vi "FTW-Actor-LocalMessage-Worker.vi"(0 "FTW-ActorInstance In":refnum<class "FTW-ActorInstance.lvclass">, 5 "Message Header":string, 7 "Message Body":string, 9 "Send Rate":dbl, 11 "error in":errorcluster, 12 "Lossless (F)":bool, 14 "max queue size (1)":i32=1) -> ()   [LabVIEW 2013, in "FTW-ActorInstance.lvclass"]
uses:
  FTW-ActorInstance.lvclass
  FTW-ActorInstance.lvclass/FTW-ActorInstance.ctl
  Message/Base/FTW-Message.lvclass
  Message/Lossy/FTW-Message-Lossy.lvclass
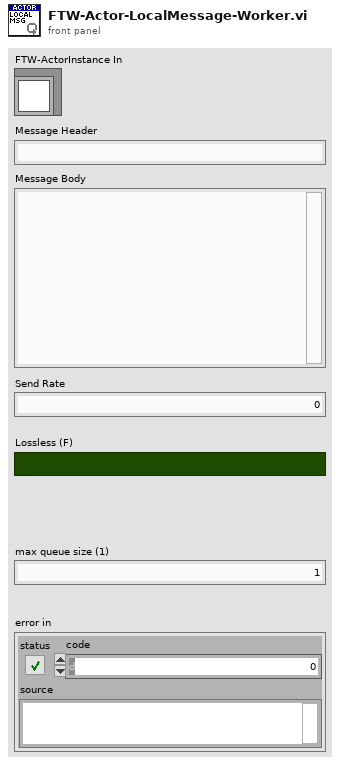
[diagram p1: front panel]
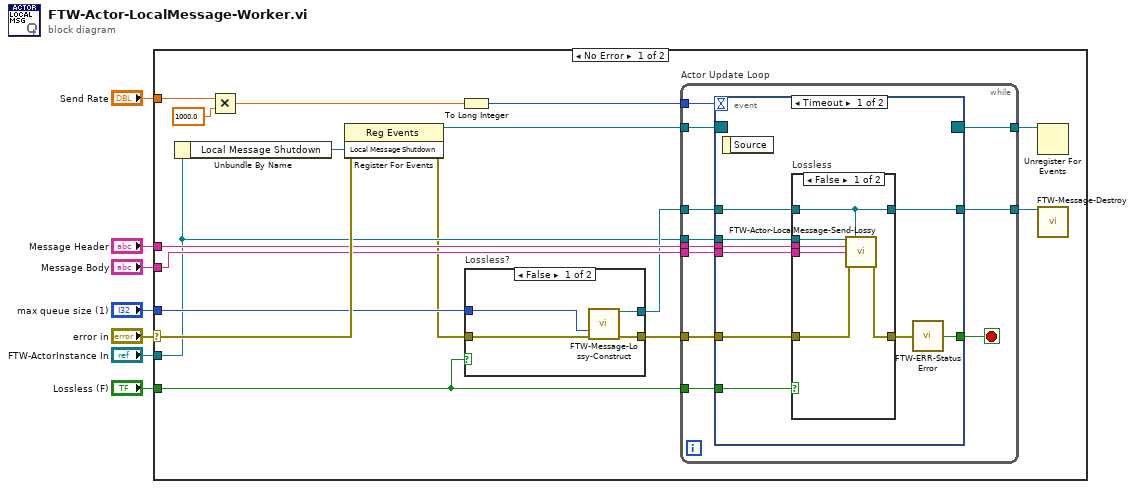
[diagram p0: block diagram]
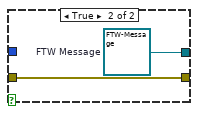
[diagram p2: hidden frame]
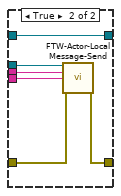
[diagram p3: hidden frame]
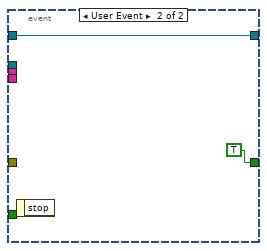
[diagram p4: hidden frame]
diagram:
  n1 = case shown="No Error" "error in" {
    selector: "error in" -> [w24 _]
    tunnel: "Message Header" -> [w23 _]
    tunnel: "Message Body" -> [w22 _]
    tunnel: "FTW-ActorInstance In" -> [w12 _]
    tunnel: "Send Rate" -> [w21 _]
    tunnel: "Lossless (F)" -> [w19 _]
    tunnel: "max queue size (1)" -> [w17 _]
    frame No Error {
      n2 = Unbundle By Name(w12) -> ("Local Message Shutdown"=w10:refnum<user-event>)
      n3 = Multiply(x=w21, y=1000.0 ("x")) -> (x*y=w15:dbl)
      n4 = register-events(error in=w24, w10) -> (reference out=w9:refnum<event-registration>, error out=w11:errorcluster)  [unwired: 1 in]
      n5 = To Long Integer(number=w15) -> (32bit integer=w13:i32)
      n6 = case "Lossless?" shown="False" w19 {
        tunnel: w11 -> [w28 w30]
        tunnel: [w27 w30] -> w20
        tunnel: [w26 w29] -> w18
        tunnel: w17 -> [w25 _]
        frame False {
          n7 = call "FTW-Message-Lossy-Construct.vi"("max queue size (1)"=w25, "error in"=w28) -> ("FTW-Message-Lossy"=w26:refnum<class "FTW-Message-Lossy.lvclass">, "error out"=w27:errorcluster)  [unwired: 12 in]
        }
        frame True {
          w29 = refnum<class "FTW-Message.lvclass"> refnum  # FTW Message
        }
      }
      n8 = while "Actor Update Loop" {
        tunnel: w12 -> [w41]
        tunnel: w23 -> [w39]
        tunnel: w22 -> [w38]
        tunnel: w13 -> [w33]
        tunnel: w20 -> [w36]
        tunnel: w19 -> [w37]
        tunnel: w18 -> [w35]
        tunnel: [w34] -> w16
        tunnel: w9 -> [w32]
        tunnel: [w31] -> w8
        stop <- w40 stop-if-true
        n9 = event shown="[0] Timeout" {
          selector: w32 -> [_ _]
          dyn-events: [_ _] -> w31
          timeout: w33 -> [_ _]
          tunnel: w41 -> [w50 _]
          tunnel: [w49 TRUE ("Error?")] -> w40
          tunnel: w39 -> [w48 _]
          tunnel: w38 -> [w47 _]
          tunnel: w37 -> [w45 _]
          tunnel: w36 -> [w44 _]
          tunnel: w35 -> [w43 w64]
          tunnel: [w42 w64] -> w34
          event Timeout {
            n10 = event-data() -> ()  [unwired: 1 in, 1 out]
            n11 = case "Lossless" shown="False" w45 {
              tunnel: w50 -> [w56 w60]
              tunnel: [w55 w61] -> w46
              tunnel: w48 -> [w54 w59]
              tunnel: w47 -> [w53 w58]
              tunnel: w44 -> [w52 w62]
              tunnel: w43 -> [w51 w57]
              tunnel: [w51 w57] -> w42
              frame False {
                n12 = call "FTW-Actor-LocalMessage-Send-Lossy.vi"("FTW-ActorInstance In"=w56, "FTW Message"=w51, "Message Header"=w54, "Message Body"=w53, "error in"=w52) -> ("error out"=w55:errorcluster)  [unwired: 10 in]
              }
              frame True {
                n13 = call "FTW-Actor-LocalMessage-Send.vi"("FTW-ActorInstance In"=w60, "Message Header"=w59, "Message Body"=w58, "error in"=w62) -> ("error out"=w61:errorcluster)  [unwired: 11 in]
              }
            }
            n14 = call "FTW-ERR-StatusError.vi"("error to check"=w46) -> ("Error?"=w49:bool)
          }
          event User Event {
            n15 = event-data() -> ()  [unwired: 1 in, 1 out]
          }
        }
      }
      n16 = Unregister For Events(event registration refnum=w8) -> ()  [unwired: 1 in, 1 out]
      n17 = call-dynamic "FTW-Message-Destroy.vi"("FTW Message"=w16) -> ()  [unwired: 14 in, 1 out]
    }
    frame Error {
    }
  }
